vi "ReadIOConfig.vi"   [LabVIEW 2012]
uses:
  <vilib>/Rock Robotics/SystemInterfaces/DIO/FPGA_DIOPWMChannel.ctl
  <vilib>/Rock Robotics/SystemInterfaces/DIO/FPGA_DIOChannel.ctl
  <vilib>/Utility/config.llb/Read Key (Boolean).vi
  <vilib>/Utility/config.llb/Read Key (I32).vi
  <vilib>/Utility/config.llb/NI_LVConfig.lvlib
types:
  T1 = typedef "NI_LVConfig.lvlib/Config Data RefNum.ctl" = refnum<k1>
  T2 = typedef "FPGA_DIOPWMChannel.ctl" = enum8{"PWM 1", "PWM 2", "PWM 3", "PWM 4", "PWM 5", "PWM 6", "PWM 7", "PWM 8", "PWM 9", "PWM 10", "Invalid"}
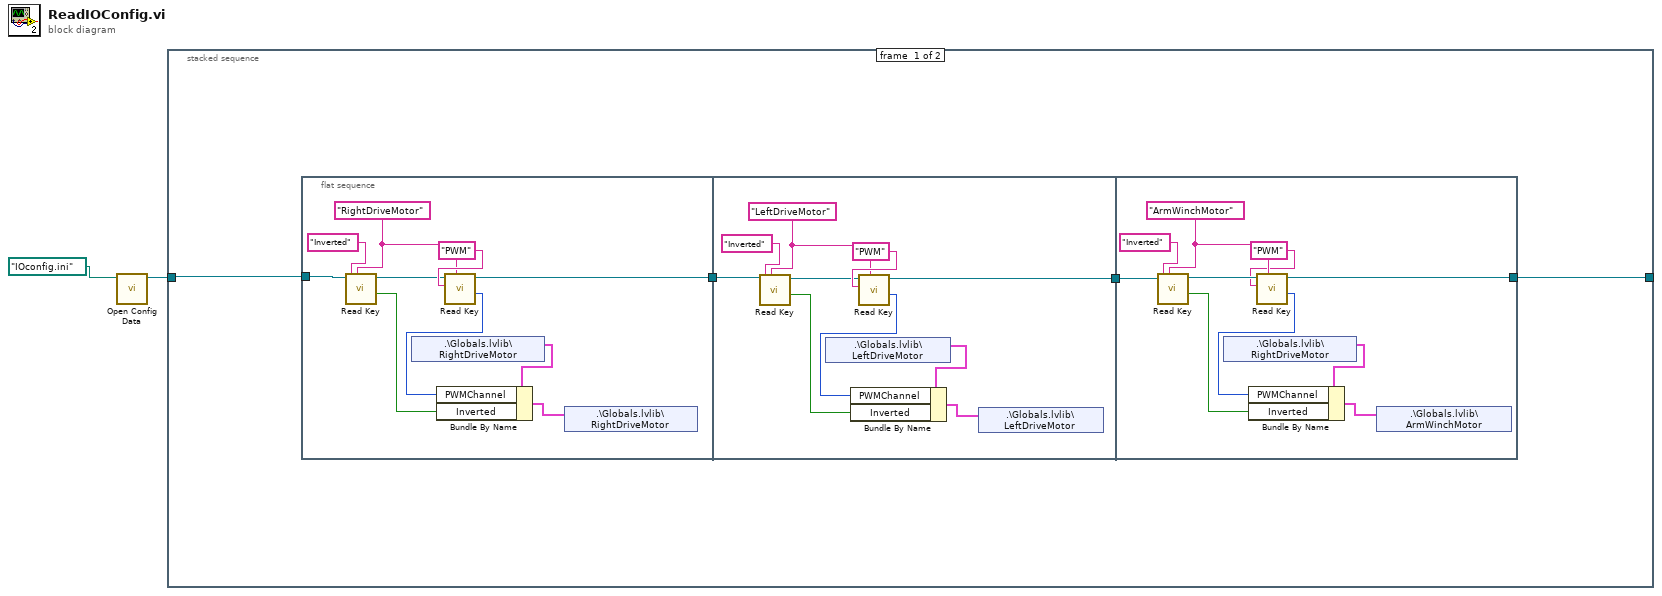
[diagram p0: block diagram]
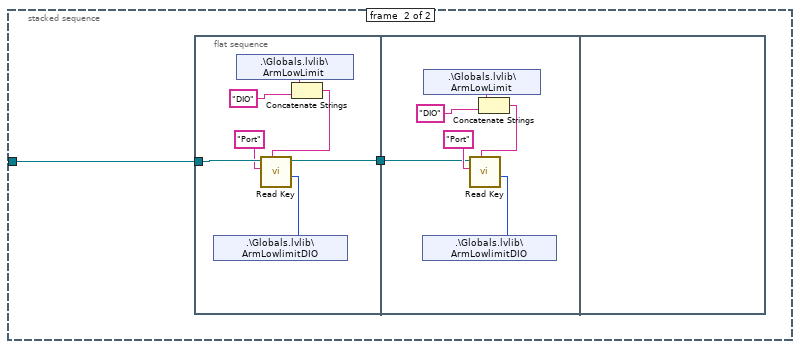
[diagram p2: hidden frame]
diagram:
  n1 = call <vilib>:"Open Config Data.vi"("configuration file path"=path "IOconfig.ini") -> ("refnum"=w1:T1)  [unwired: 8 in, 2 out]
  n2 = stacked-sequence {
    tunnel: w1 -> [w5 w38]
    tunnel: [w3 _] -> _
    frame #0 {
      n3 = flat-sequence {
        tunnel: w5 -> [w16]
        tunnel: [w7] -> w6
        tunnel: w6 -> [w18]
        tunnel: [w17] -> w4
        tunnel: w4 -> [w28]
        tunnel: [w27] -> w3
        frame #0 {
          w11 = "RightDriveMotor"
          n4 = call-poly <vilib>:"Read Key.vi"("section"=w11, "key"="Inverted", "refnum"=w16) -> ("value"=w8:bool, "refnum out"=w10:T1)  [unwired: 5 in, 2 out]
          n5 = shared-variable ".\\Globals.lvlib\\RightDriveMotor"() -> (w15:cluster{"PWMChannel":T2, "Inverted":bool})  [unwired: 1 in, 1 out]
          n6 = call-poly <vilib>:"Read Key.vi"("section"=w11, "key"="PWM", "refnum"=w10) -> ("value"=w9:i32, "refnum out"=w7:T1)  [unwired: 5 in, 2 out]
          n7 = Bundle By Name(cluster=w15, "PWMChannel"=w9, "Inverted"=w8) -> (w14:cluster{"PWMChannel":T2, "Inverted":bool})
          n8 = shared-variable ".\\Globals.lvlib\\RightDriveMotor"(w14) -> ()  [unwired: 1 in, 1 out]
        }
        frame #1 {
          w22 = "LeftDriveMotor"
          n9 = call-poly <vilib>:"Read Key.vi"("section"=w22, "key"="Inverted", "refnum"=w18) -> ("value"=w19:bool, "refnum out"=w21:T1)  [unwired: 5 in, 2 out]
          n10 = shared-variable ".\\Globals.lvlib\\LeftDriveMotor"() -> (w26:cluster{"PWMChannel":T2, "Inverted":bool})  [unwired: 1 in, 1 out]
          n11 = call-poly <vilib>:"Read Key.vi"("section"=w22, "key"="PWM", "refnum"=w21) -> ("value"=w20:i32, "refnum out"=w17:T1)  [unwired: 5 in, 2 out]
          n12 = Bundle By Name(cluster=w26, "PWMChannel"=w20, "Inverted"=w19) -> (w25:cluster{"PWMChannel":T2, "Inverted":bool})
          n13 = shared-variable ".\\Globals.lvlib\\LeftDriveMotor"(w25) -> ()  [unwired: 1 in, 1 out]
        }
        frame #2 {
          w33 = "ArmWinchMotor"
          n14 = call-poly <vilib>:"Read Key.vi"("section"=w33, "key"="Inverted", "refnum"=w28) -> ("value"=w36:bool, "refnum out"=w34:T1)  [unwired: 5 in, 2 out]
          n15 = shared-variable ".\\Globals.lvlib\\RightDriveMotor"() -> (w29:cluster{"PWMChannel":T2, "Inverted":bool})  [unwired: 1 in, 1 out]
          n16 = call-poly <vilib>:"Read Key.vi"("section"=w33, "key"="PWM", "refnum"=w34) -> ("value"=w35:i32, "refnum out"=w27:T1)  [unwired: 5 in, 2 out]
          n17 = Bundle By Name(cluster=w29, "PWMChannel"=w35, "Inverted"=w36) -> (w30:cluster{"PWMChannel":T2, "Inverted":bool})
          n18 = shared-variable ".\\Globals.lvlib\\ArmWinchMotor"(w30) -> ()  [unwired: 1 in, 1 out]
        }
      }
    }
    frame #1 {
      n19 = flat-sequence {
        tunnel: w38 -> [w45]
        tunnel: [w42] -> w37
        tunnel: w37 -> [w49]
        frame #0 {
          n20 = shared-variable ".\\Globals.lvlib\\ArmLowLimit"() -> (w41:string)  [unwired: 1 in, 1 out]
          n21 = Concatenate Strings(w41, "DIO") -> (w39:string)
          n22 = call-poly <vilib>:"Read Key.vi"("section"=w39, "key"="Port", "refnum"=w45) -> ("value"=w43:i32, "refnum out"=w42:T1)  [unwired: 5 in, 2 out]
          n23 = shared-variable ".\\Globals.lvlib\\ArmLowlimitDIO"(w43) -> ()  [unwired: 1 in, 1 out]
        }
        frame #1 {
          n24 = shared-variable ".\\Globals.lvlib\\ArmLowLimit"() -> (w47:string)  [unwired: 1 in, 1 out]
          n25 = Concatenate Strings(w47, "DIO") -> (w46:string)
          n26 = call-poly <vilib>:"Read Key.vi"("section"=w46, "key"="Port", "refnum"=w49) -> ("value"=w50:i32)  [unwired: 5 in, 3 out]
          n27 = shared-variable ".\\Globals.lvlib\\ArmLowlimitDIO"(w50) -> ()  [unwired: 1 in, 1 out]
        }
        frame #2 {
        }
      }
    }
  }
